vi "骰寶.vi"() -> ()   [LabVIEW 2014]
panel:
  in  "Listbox 2":i32[](listbox)
  in  "Listbox 3":i32[](listbox)
  in  "Listbox":i32[](listbox)
  in  "遊戲開始":bool
  out "總共賺取/賠掉金額":i32
  out "經歷輪數":i32
  out "此輪賺取/賠掉金額":i32
  out "賭金金額":i32
  out "Boolean":T1
  in  "Cluster 7":T2={"Color Box 4"=16448250, "Boolean 5"=FALSE, "Boolean 11"=FALSE, "Boolean 12"=FALSE, "Boolean 13"=FALSE, "Boolean 14"=FALSE, "Boolean 15"=FALSE}
  in  "Cluster 6":T3={"Color Box"=16777215, "Boolean 4"=FALSE, "Boolean 5"=FALSE, "Boolean 6"=FALSE, "Boolean 7"=FALSE, "Boolean 8"=FALSE}
  in  "Cluster 5":T4={"Color Box 2"=16777215, "Boolean 3"=FALSE, "Boolean 4"=FALSE, "Boolean 6"=FALSE, "Boolean 5"=FALSE}
  in  "Cluster 4":T5={"Color Box 2"=16777215, "Boolean"=FALSE, "Boolean 3"=FALSE, "Boolean 2"=FALSE}
  in  "Cluster 3":T6={"Color Box"=16777215, "Boolean"=FALSE, "Boolean 2"=FALSE}
  in  "Cluster 2":T7={"Color Box"=16777215, "Boolean"=FALSE}
  in  "下注金額":i32=10 min=10 max=50
  out "Enum":enum16{"3", "2", "1"}(ring)=enum."2"
  out "骰子點數":i32
  out "比較值3":i32
  out "比較值2":i32
  out "比較值1":i32
  in  "退出比賽":bool
  in  "下好離手":bool
  in  "進行下一輪":bool
  in  "下注盤":T8
  # "遊戲介紹:"
  # "遊戲操作:"
  # "注意事項:"
  # "以上說明都看完沒問題的話，\n就可以按下遊戲開始開始遊玩囉!\n                        ↓"
  # "骰子點數"
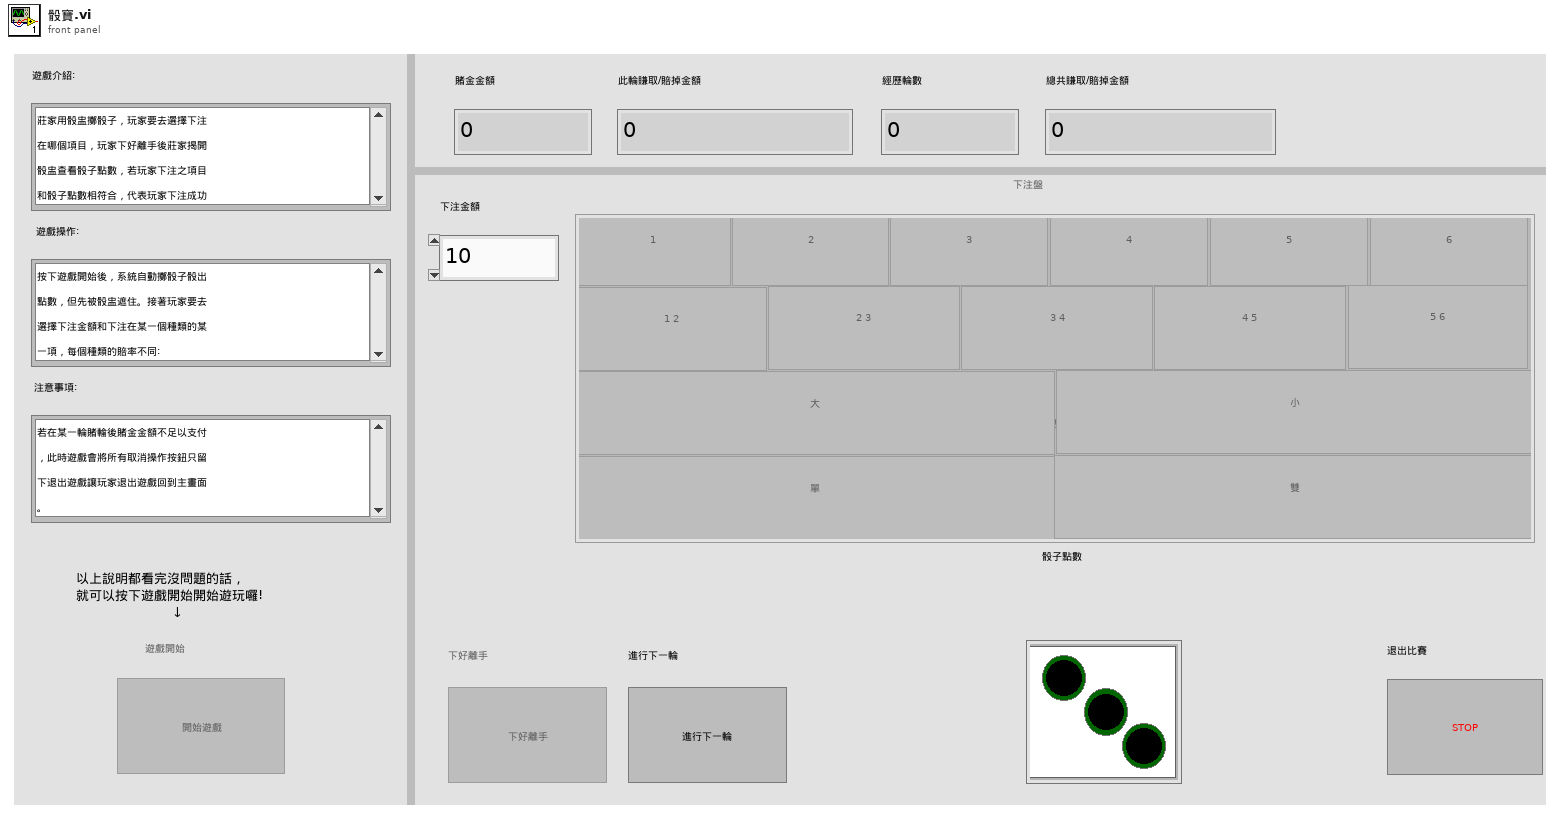
[diagram p1: front panel]
types:
  T1 = typedef "骰盅.ctl" = bool
  T2 = typedef "點數六.ctl" = cluster{"Color Box 4":u32, "Boolean 5":bool, "Boolean 11":bool, "Boolean 12":bool, "Boolean 13":bool, "Boolean 14":bool, "Boolean 15":bool}
  T3 = typedef "き.ctl" = cluster{"Color Box":u32, "Boolean 4":bool, "Boolean 5":bool, "Boolean 6":bool, "Boolean 7":bool, "Boolean 8":bool}
  T4 = typedef "點數四.ctl" = cluster{"Color Box 2":u32, "Boolean 3":bool, "Boolean 4":bool, "Boolean 6":bool, "Boolean 5":bool}
  T5 = typedef "點數三.ctl" = cluster{"Color Box 2":u32, "Boolean":bool, "Boolean 3":bool, "Boolean 2":bool}
  T6 = typedef "點數二.ctl" = cluster{"Color Box":u32, "Boolean":bool, "Boolean 2":bool}
  T7 = typedef "點數一.ctl" = cluster{"Color Box":u32, "Boolean":bool}
  T8 = cluster{" 單":bool, "雙":bool, "大":bool, "小 ":bool, "1 2":bool, "2 3":bool, "3 4":bool, "4 5":bool, "5 6":bool, "1":bool, "2":bool, "3":bool, "4 ":bool, "5":bool, "6":bool}
  T9 = enum16{"restart", "display dice's number and compare 3", "display dice's number and compare 2", "display dice's number and compare 1", "Get out of hand", "player select item", "throw dice(not display)", "wait start button press", "init"}
  T10 = enum8{"Enabled", "Disabled", "Disabled and Grayed Out"}
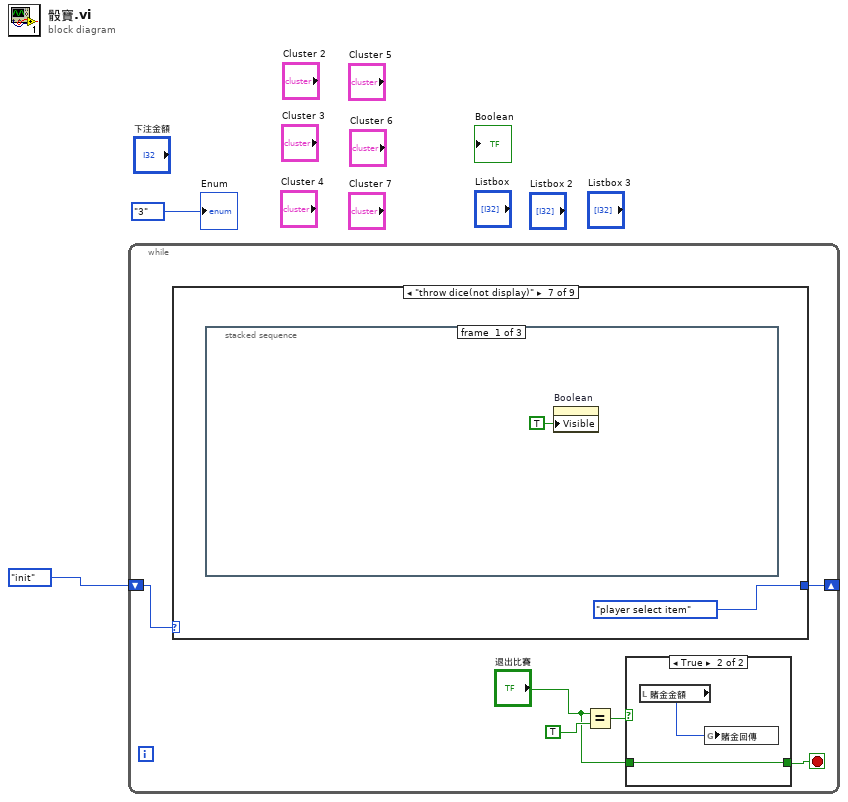
[diagram p0: block diagram]
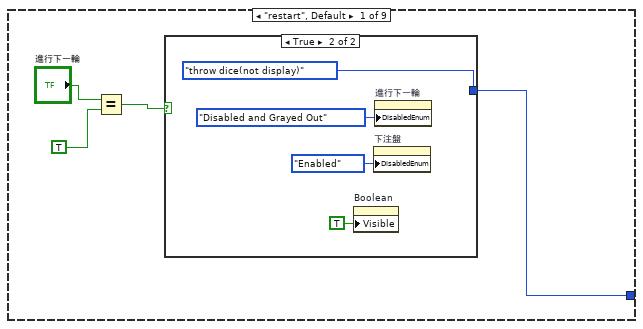
[diagram p3: hidden frame]
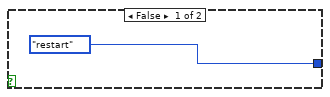
[diagram p4: hidden frame]
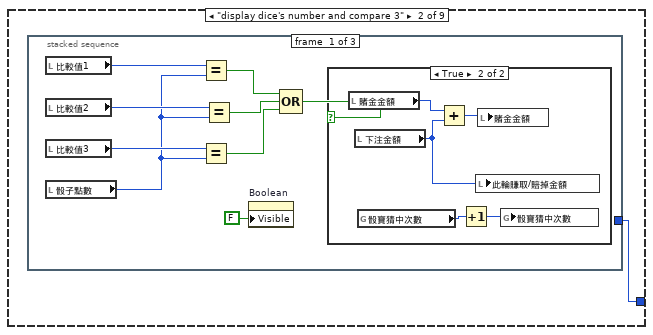
[diagram p5: hidden frame]
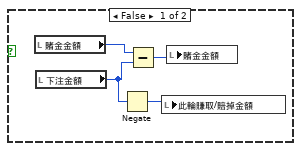
[diagram p6: hidden frame]
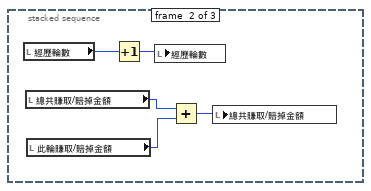
[diagram p7: hidden frame]
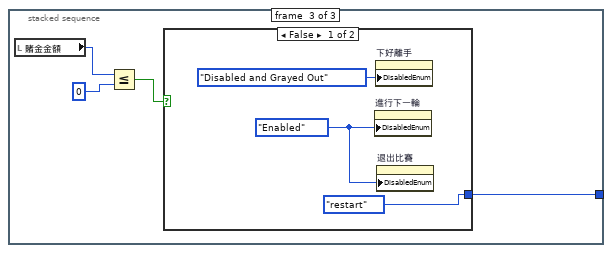
[diagram p8: hidden frame]
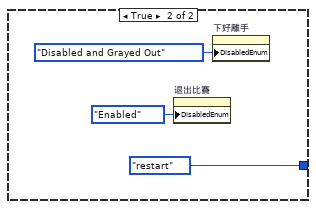
[diagram p9: hidden frame]
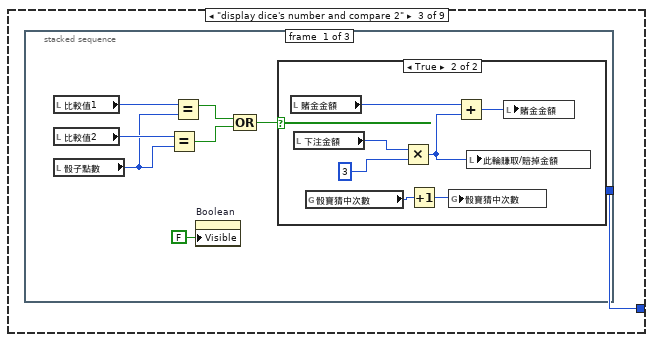
[diagram p10: hidden frame]
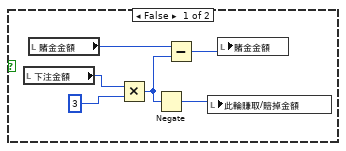
[diagram p11: hidden frame]
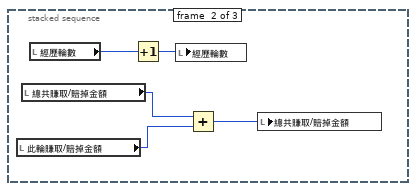
[diagram p12: hidden frame]
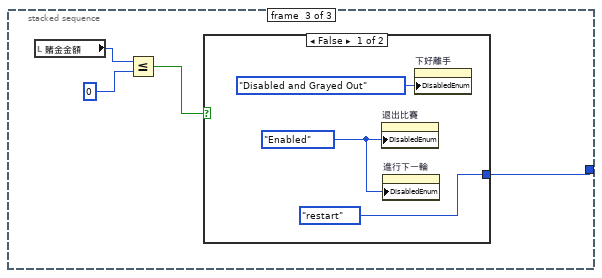
[diagram p13: hidden frame]
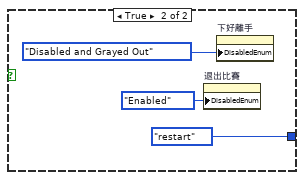
[diagram p14: hidden frame]
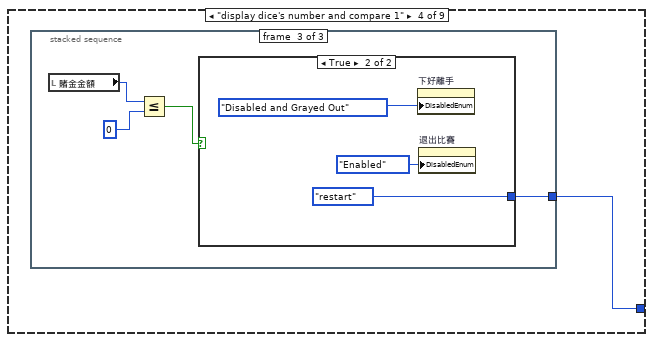
[diagram p15: hidden frame]
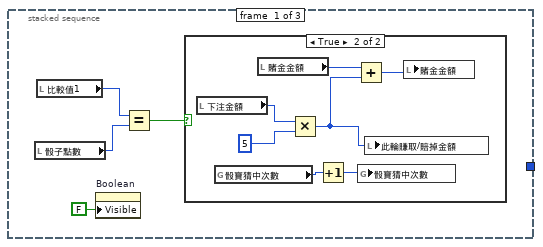
[diagram p16: hidden frame]
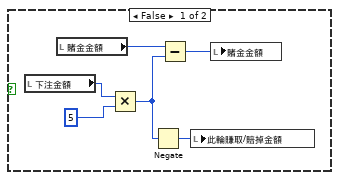
[diagram p17: hidden frame]
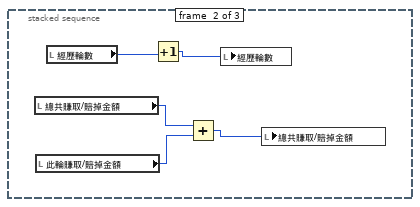
[diagram p18: hidden frame]
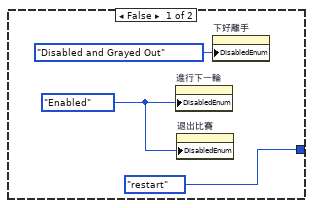
[diagram p19: hidden frame]
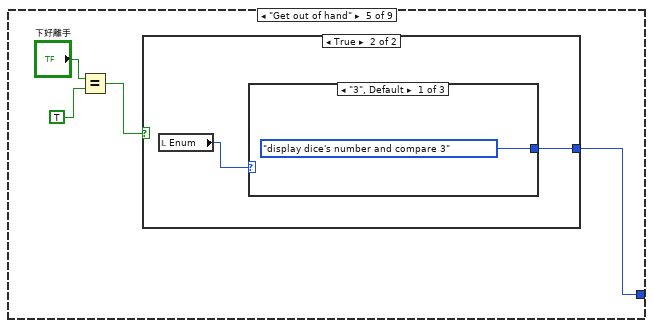
[diagram p20: hidden frame]
diagram:
  n1 = while {
    shift-right: [w7] -> _
    shift-left: T9."init" -> [w8]
    stop <- w3 stop-if-true
    n2 = case shown="\"throw dice(not display)\"" w8 {
      tunnel: [w12 w21 w55 w91 w124 w134 T9."player select item" w249 T9."wait start button press"] -> w7
      frame "restart", Default {
        n3 = Equal?(x="進行下一輪", y=TRUE) -> (x = y?=w15:bool)
        n4 = case shown="True" w15 {
          tunnel: [T9."restart" T9."throw dice(not display)"] -> w12
          frame False {
          }
          frame True {
            n5 = property on="Boolean" class="Bool (strict)"("Visible"=TRUE) -> ()  [unwired: 2 in, 2 out]
            n6 = property on="下注盤" class="Clust"("DisabledEnum"=T10."Enabled" ("Disabled")) -> ()  [unwired: 2 in, 2 out]
            n7 = property on="進行下一輪" class="Bool"("DisabledEnum"=T10."Disabled and Grayed Out" ("Disabled")) -> ()  [unwired: 2 in, 2 out]
          }
        }
      }
      frame "display dice's number and compare 3" {
        n8 = stacked-sequence {
          tunnel: [_ _ w45] -> w21
          frame #0 {
            n9 = local read "比較值1"() -> (w30:i32)
            n10 = local read "比較值2"() -> (w29:i32)
            n11 = local read "比較值3"() -> (w28:i32)
            n12 = local read "骰子點數"() -> (w27:i32)
            n13 = Equal?(x=w30, y=w27) -> (x = y?=w26:bool)
            n14 = Equal?(x=w28, y=w27) -> (x = y?=w24:bool)
            n15 = Equal?(x=w29, y=w27) -> (x = y?=w25:bool)
            n16 = property on="Boolean" class="Bool (strict)"("Visible"=FALSE) -> ()  [unwired: 2 in, 2 out]
            n17 = Compound Arithmetic op=OR(w26, w25, w24) -> (w23:bool)
            n18 = case shown="True" w23 {
              frame False {
                n19 = local read "賭金金額"() -> (w34:i32)
                n20 = local read "下注金額"() -> (w31:i32)
                n21 = Negate(x=w31) -> (-x=w32:i32)
                n22 = Subtract(x=w34, y=w31) -> (x-y=w33:i32)
                n23 = local write "此輪賺取/賠掉金額"(w32) -> ()
                n24 = local write "賭金金額"(w33) -> ()
              }
              frame True {
                n25 = local read "賭金金額"() -> (w39:i32)
                n26 = local read "下注金額"() -> (w37:i32)
                n27 = global read "global variable-骰寶猜中次數.vi" "骰寶猜中次數"() -> (w36:i32)
                n28 = Add(x=w39, y=w37) -> (x+y=w38:i32)
                n29 = Increment(x=w36) -> (x+1=w35:i32)
                n30 = local write "此輪賺取/賠掉金額"(w37) -> ()
                n31 = local write "賭金金額"(w38) -> ()
                n32 = global write "global variable-骰寶猜中次數.vi" "骰寶猜中次數"(w35) -> ()
              }
            }
          }
          frame #1 {
            n33 = local read "經歷輪數"() -> (w44:i32)
            n34 = local read "總共賺取/賠掉金額"() -> (w42:i32)
            n35 = local read "此輪賺取/賠掉金額"() -> (w41:i32)
            n36 = Increment(x=w44) -> (x+1=w43:i32)
            n37 = local write "經歷輪數"(w43) -> ()
            n38 = Add(x=w42, y=w41) -> (x+y=w40:i32)
            n39 = local write "總共賺取/賠掉金額"(w40) -> ()
          }
          frame #2 {
            n40 = local read "賭金金額"() -> (w48:i32)
            n41 = Less Or Equal?(x=w48, y=0) -> (x <= y?=w46:bool)
            n42 = case shown="False" w46 {
              tunnel: [T9."restart" T9."restart"] -> w45
              frame False {
                w50 = T10."Enabled" ("Disabled")
                n43 = property on="進行下一輪" class="Bool"("DisabledEnum"=w50) -> ()  [unwired: 2 in, 2 out]
                n44 = property on="下好離手" class="Bool"("DisabledEnum"=T10."Disabled and Grayed Out" ("Disabled")) -> ()  [unwired: 2 in, 2 out]
                n45 = property on="退出比賽" class="Bool"("DisabledEnum"=w50) -> ()  [unwired: 2 in, 2 out]
              }
              frame True {
                n46 = property on="退出比賽" class="Bool"("DisabledEnum"=T10."Enabled" ("Disabled")) -> ()  [unwired: 2 in, 2 out]
                n47 = property on="下好離手" class="Bool"("DisabledEnum"=T10."Disabled and Grayed Out" ("Disabled")) -> ()  [unwired: 2 in, 2 out]
              }
            }
          }
        }
      }
      frame "display dice's number and compare 2" {
        n48 = stacked-sequence {
          tunnel: [_ _ w81] -> w55
          frame #0 {
            n49 = local read "比較值1"() -> (w62:i32)
            n50 = local read "比較值2"() -> (w61:i32)
            n51 = local read "骰子點數"() -> (w60:i32)
            n52 = Equal?(x=w61, y=w60) -> (x = y?=w58:bool)
            n53 = Equal?(x=w62, y=w60) -> (x = y?=w59:bool)
            n54 = property on="Boolean" class="Bool (strict)"("Visible"=FALSE) -> ()  [unwired: 2 in, 2 out]
            n55 = Compound Arithmetic op=OR(w59, w58) -> (w57:bool)
            n56 = case shown="True" w57 {
              frame False {
                n57 = local read "下注金額"() -> (w68:i32)
                n58 = local read "賭金金額"() -> (w66:i32)
                n59 = Multiply(x=w68, y=3) -> (x*y=w63:i32)
                n60 = Negate(x=w63) -> (-x=w64:i32)
                n61 = Subtract(x=w66, y=w63) -> (x-y=w65:i32)
                n62 = local write "此輪賺取/賠掉金額"(w64) -> ()
                n63 = local write "賭金金額"(w65) -> ()
              }
              frame True {
                n64 = local read "賭金金額"() -> (w73:i32)
                n65 = local read "下注金額"() -> (w75:i32)
                n66 = global read "global variable-骰寶猜中次數.vi" "骰寶猜中次數"() -> (w69:i32)
                n67 = Multiply(x=w75, y=3) -> (x*y=w71:i32)
                n68 = Increment(x=w69) -> (x+1=w70:i32)
                n69 = global write "global variable-骰寶猜中次數.vi" "骰寶猜中次數"(w70) -> ()
                n70 = Add(x=w73, y=w71) -> (x+y=w72:i32)
                n71 = local write "此輪賺取/賠掉金額"(w71) -> ()
                n72 = local write "賭金金額"(w72) -> ()
              }
            }
          }
          frame #1 {
            n73 = local read "此輪賺取/賠掉金額"() -> (w77:i32)
            n74 = local read "總共賺取/賠掉金額"() -> (w78:i32)
            n75 = local read "經歷輪數"() -> (w80:i32)
            n76 = Increment(x=w80) -> (x+1=w79:i32)
            n77 = local write "經歷輪數"(w79) -> ()
            n78 = Add(x=w78, y=w77) -> (x+y=w76:i32)
            n79 = local write "總共賺取/賠掉金額"(w76) -> ()
          }
          frame #2 {
            n80 = local read "賭金金額"() -> (w84:i32)
            n81 = Less Or Equal?(x=w84, y=0) -> (x <= y?=w82:bool)
            n82 = case shown="False" w82 {
              tunnel: [T9."restart" T9."restart"] -> w81
              frame False {
                w87 = T10."Enabled" ("Disabled")
                n83 = property on="退出比賽" class="Bool"("DisabledEnum"=w87) -> ()  [unwired: 2 in, 2 out]
                n84 = property on="進行下一輪" class="Bool"("DisabledEnum"=w87) -> ()  [unwired: 2 in, 2 out]
                n85 = property on="下好離手" class="Bool"("DisabledEnum"=T10."Disabled and Grayed Out" ("Disabled")) -> ()  [unwired: 2 in, 2 out]
              }
              frame True {
                n86 = property on="退出比賽" class="Bool"("DisabledEnum"=T10."Enabled" ("Disabled")) -> ()  [unwired: 2 in, 2 out]
                n87 = property on="下好離手" class="Bool"("DisabledEnum"=T10."Disabled and Grayed Out" ("Disabled")) -> ()  [unwired: 2 in, 2 out]
              }
            }
          }
        }
      }
      frame "display dice's number and compare 1" {
        n88 = stacked-sequence {
          tunnel: [_ _ w114] -> w91
          frame #0 {
            n89 = local read "骰子點數"() -> (w95:i32)
            n90 = local read "比較值1"() -> (w94:i32)
            n91 = property on="Boolean" class="Bool (strict)"("Visible"=FALSE) -> ()  [unwired: 2 in, 2 out]
            n92 = Equal?(x=w94, y=w95) -> (x = y?=w93:bool)
            n93 = case shown="True" w93 {
              frame False {
                n94 = local read "下注金額"() -> (w101:i32)
                n95 = local read "賭金金額"() -> (w99:i32)
                n96 = Multiply(x=w101, y=5) -> (x*y=w96:i32)
                n97 = Negate(x=w96) -> (-x=w97:i32)
                n98 = Subtract(x=w99, y=w96) -> (x-y=w98:i32)
                n99 = local write "此輪賺取/賠掉金額"(w97) -> ()
                n100 = local write "賭金金額"(w98) -> ()
              }
              frame True {
                n101 = local read "下注金額"() -> (w108:i32)
                n102 = global read "global variable-骰寶猜中次數.vi" "骰寶猜中次數"() -> (w102:i32)
                n103 = local read "賭金金額"() -> (w106:i32)
                n104 = Multiply(x=w108, y=5) -> (x*y=w104:i32)
                n105 = Increment(x=w102) -> (x+1=w103:i32)
                n106 = Add(x=w106, y=w104) -> (x+y=w105:i32)
                n107 = global write "global variable-骰寶猜中次數.vi" "骰寶猜中次數"(w103) -> ()
                n108 = local write "此輪賺取/賠掉金額"(w104) -> ()
                n109 = local write "賭金金額"(w105) -> ()
              }
            }
          }
          frame #1 {
            n110 = local read "總共賺取/賠掉金額"() -> (w111:i32)
            n111 = local read "此輪賺取/賠掉金額"() -> (w110:i32)
            n112 = local read "經歷輪數"() -> (w113:i32)
            n113 = Increment(x=w113) -> (x+1=w112:i32)
            n114 = Add(x=w111, y=w110) -> (x+y=w109:i32)
            n115 = local write "經歷輪數"(w112) -> ()
            n116 = local write "總共賺取/賠掉金額"(w109) -> ()
          }
          frame #2 {
            n117 = local read "賭金金額"() -> (w117:i32)
            n118 = Less Or Equal?(x=w117, y=0) -> (x <= y?=w115:bool)
            n119 = case shown="True" w115 {
              tunnel: [T9."restart" T9."restart"] -> w114
              frame False {
                w120 = T10."Enabled" ("Disabled")
                n120 = property on="進行下一輪" class="Bool"("DisabledEnum"=w120) -> ()  [unwired: 2 in, 2 out]
                n121 = property on="退出比賽" class="Bool"("DisabledEnum"=w120) -> ()  [unwired: 2 in, 2 out]
                n122 = property on="下好離手" class="Bool"("DisabledEnum"=T10."Disabled and Grayed Out" ("Disabled")) -> ()  [unwired: 2 in, 2 out]
              }
              frame True {
                n123 = property on="下好離手" class="Bool"("DisabledEnum"=T10."Disabled and Grayed Out" ("Disabled")) -> ()  [unwired: 2 in, 2 out]
                n124 = property on="退出比賽" class="Bool"("DisabledEnum"=T10."Enabled" ("Disabled")) -> ()  [unwired: 2 in, 2 out]
              }
            }
          }
        }
      }
      frame "Get out of hand" {
        n125 = Equal?(x="下好離手", y=TRUE) -> (x = y?=w126:bool)
        n126 = case shown="True" w126 {
          tunnel: [T9."Get out of hand" w129] -> w124
          frame False {
          }
          frame True {
            n127 = local read "Enum"() -> (w130:enum16{"3", "2", "1"})
            n128 = case shown="\"3\", Default" w130 {
              tunnel: [T9."display dice's number and compare 3" T9."display dice's number and compare 2" T9."display dice's number and compare 1"] -> w129
              frame "3", Default {
              }
              frame "2" {
              }
              frame "1" {
              }
            }
          }
        }
      }
      frame "player select item" {
        n129 = Cluster To Array(cluster="下注盤") -> (array=w136:bool[])
        n130 = Search 1D Array(1D array=w136, element=TRUE) -> (index of element=w138:i32)  [unwired: 1 in]
        n131 = case shown="0" w138 {
          tunnel: [T9."player select item" T9."Get out of hand" T9."Get out of hand" T9."Get out of hand" T9."Get out of hand" T9."Get out of hand" T9."Get out of hand" T9."Get out of hand" T9."Get out of hand" T9."Get out of hand" T9."Get out of hand" T9."Get out of hand" T9."Get out of hand" T9."Get out of hand" T9."Get out of hand" T9."Get out of hand"] -> w134
          frame -1, Default {
          }
          frame 0 {
            n132 = local write "比較值2"(3 ("比較值2")) -> ()
            n133 = local write "比較值3"(5 ("比較值3")) -> ()
            n134 = local write "比較值1"(1) -> ()
            n135 = local write "Enum"(enum16{"3", "2", "1"}."3" ("Enum")) -> ()
            n136 = property on="下好離手" class="Bool"("DisabledEnum"=T10."Enabled" ("Disabled")) -> ()  [unwired: 2 in, 2 out]
            n137 = property on="下注盤" class="Clust"("DisabledEnum"=T10."Disabled and Grayed Out" ("Disabled")) -> ()  [unwired: 2 in, 2 out]
          }
          frame 1 {
            n138 = local write "比較值3"(6 ("比較值3")) -> ()
            n139 = local write "比較值2"(4 ("比較值2")) -> ()
            n140 = local write "比較值1"(2 ("比較值1")) -> ()
            n141 = local write "Enum"(enum16{"3", "2", "1"}."3" ("Enum")) -> ()
            n142 = property on="下好離手" class="Bool"("DisabledEnum"=T10."Enabled" ("Disabled")) -> ()  [unwired: 2 in, 2 out]
            n143 = property on="下注盤" class="Clust"("DisabledEnum"=T10."Disabled and Grayed Out" ("Disabled")) -> ()  [unwired: 2 in, 2 out]
          }
          frame 2 {
            n144 = local write "比較值3"(4 ("比較值3")) -> ()
            n145 = local write "比較值1"(6 ("比較值1")) -> ()
            n146 = local write "比較值2"(5 ("比較值2")) -> ()
            n147 = local write "Enum"(enum16{"3", "2", "1"}."3" ("Enum")) -> ()
            n148 = property on="下好離手" class="Bool"("DisabledEnum"=T10."Enabled" ("Disabled")) -> ()  [unwired: 2 in, 2 out]
            n149 = property on="下注盤" class="Clust"("DisabledEnum"=T10."Disabled and Grayed Out" ("Disabled")) -> ()  [unwired: 2 in, 2 out]
          }
          frame 3 {
            n150 = local write "比較值2"(2 ("比較值2")) -> ()
            n151 = local write "比較值3"(1 ("比較值3")) -> ()
            n152 = local write "比較值1"(3 ("比較值1")) -> ()
            n153 = local write "Enum"(enum16{"3", "2", "1"}."3" ("Enum")) -> ()
            n154 = property on="下好離手" class="Bool"("DisabledEnum"=T10."Enabled" ("Disabled")) -> ()  [unwired: 2 in, 2 out]
            n155 = property on="下注盤" class="Clust"("DisabledEnum"=T10."Disabled and Grayed Out" ("Disabled")) -> ()  [unwired: 2 in, 2 out]
          }
          frame 4 {
            n156 = local write "比較值1"(1 ("比較值1")) -> ()
            n157 = local write "比較值2"(2 ("比較值2")) -> ()
            n158 = local write "Enum"(enum16{"3", "2", "1"}."2" ("Enum")) -> ()
            n159 = property on="下好離手" class="Bool"("DisabledEnum"=T10."Enabled" ("Disabled")) -> ()  [unwired: 2 in, 2 out]
            n160 = property on="下注盤" class="Clust"("DisabledEnum"=T10."Disabled and Grayed Out" ("Disabled")) -> ()  [unwired: 2 in, 2 out]
          }
          frame 5 {
            n161 = local write "比較值1"(2 ("比較值1")) -> ()
            n162 = local write "比較值2"(3 ("比較值2")) -> ()
            n163 = local write "Enum"(enum16{"3", "2", "1"}."2" ("Enum")) -> ()
            n164 = property on="下好離手" class="Bool"("DisabledEnum"=T10."Enabled" ("Disabled")) -> ()  [unwired: 2 in, 2 out]
            n165 = property on="下注盤" class="Clust"("DisabledEnum"=T10."Disabled and Grayed Out" ("Disabled")) -> ()  [unwired: 2 in, 2 out]
          }
          frame 6 {
            n166 = local write "比較值1"(3 ("比較值1")) -> ()
            n167 = local write "比較值2"(4 ("比較值2")) -> ()
            n168 = local write "Enum"(enum16{"3", "2", "1"}."2" ("Enum")) -> ()
            n169 = property on="下好離手" class="Bool"("DisabledEnum"=T10."Enabled" ("Disabled")) -> ()  [unwired: 2 in, 2 out]
            n170 = property on="下注盤" class="Clust"("DisabledEnum"=T10."Disabled and Grayed Out" ("Disabled")) -> ()  [unwired: 2 in, 2 out]
          }
          frame 7 {
            n171 = local write "比較值1"(4 ("比較值1")) -> ()
            n172 = local write "比較值2"(5 ("比較值2")) -> ()
            n173 = local write "Enum"(enum16{"3", "2", "1"}."2" ("Enum")) -> ()
            n174 = property on="下好離手" class="Bool"("DisabledEnum"=T10."Enabled" ("Disabled")) -> ()  [unwired: 2 in, 2 out]
            n175 = property on="下注盤" class="Clust"("DisabledEnum"=T10."Disabled and Grayed Out" ("Disabled")) -> ()  [unwired: 2 in, 2 out]
          }
          frame 8 {
            n176 = local write "比較值2"(6 ("比較值2")) -> ()
            n177 = local write "比較值1"(5 ("比較值1")) -> ()
            n178 = local write "Enum"(enum16{"3", "2", "1"}."2" ("Enum")) -> ()
            n179 = property on="下好離手" class="Bool"("DisabledEnum"=T10."Enabled" ("Disabled")) -> ()  [unwired: 2 in, 2 out]
            n180 = property on="下注盤" class="Clust"("DisabledEnum"=T10."Disabled and Grayed Out" ("Disabled")) -> ()  [unwired: 2 in, 2 out]
          }
          frame 9 {
            n181 = local write "比較值1"(1 ("比較值1")) -> ()
            n182 = local write "Enum"(enum16{"3", "2", "1"}."1" ("Enum")) -> ()
            n183 = property on="下好離手" class="Bool"("DisabledEnum"=T10."Enabled" ("Disabled")) -> ()  [unwired: 2 in, 2 out]
            n184 = property on="下注盤" class="Clust"("DisabledEnum"=T10."Disabled and Grayed Out" ("Disabled")) -> ()  [unwired: 2 in, 2 out]
          }
          frame 10 {
            n185 = local write "比較值1"(2 ("比較值1")) -> ()
            n186 = local write "Enum"(enum16{"3", "2", "1"}."1" ("Enum")) -> ()
            n187 = property on="下好離手" class="Bool"("DisabledEnum"=T10."Enabled" ("Disabled")) -> ()  [unwired: 2 in, 2 out]
            n188 = property on="下注盤" class="Clust"("DisabledEnum"=T10."Disabled and Grayed Out" ("Disabled")) -> ()  [unwired: 2 in, 2 out]
          }
          frame 11 {
            n189 = local write "比較值1"(3 ("比較值1")) -> ()
            n190 = local write "Enum"(enum16{"3", "2", "1"}."1" ("Enum")) -> ()
            n191 = property on="下好離手" class="Bool"("DisabledEnum"=T10."Enabled" ("Disabled")) -> ()  [unwired: 2 in, 2 out]
            n192 = property on="下注盤" class="Clust"("DisabledEnum"=T10."Disabled and Grayed Out" ("Disabled")) -> ()  [unwired: 2 in, 2 out]
          }
          frame 12 {
            n193 = local write "比較值1"(4 ("比較值1")) -> ()
            n194 = local write "Enum"(enum16{"3", "2", "1"}."1" ("Enum")) -> ()
            n195 = property on="下好離手" class="Bool"("DisabledEnum"=T10."Enabled" ("Disabled")) -> ()  [unwired: 2 in, 2 out]
            n196 = property on="下注盤" class="Clust"("DisabledEnum"=T10."Disabled and Grayed Out" ("Disabled")) -> ()  [unwired: 2 in, 2 out]
          }
          frame 13 {
            n197 = local write "比較值1"(5 ("比較值1")) -> ()
            n198 = local write "Enum"(enum16{"3", "2", "1"}."1" ("Enum")) -> ()
            n199 = property on="下好離手" class="Bool"("DisabledEnum"=T10."Enabled" ("Disabled")) -> ()  [unwired: 2 in, 2 out]
            n200 = property on="下注盤" class="Clust"("DisabledEnum"=T10."Disabled and Grayed Out" ("Disabled")) -> ()  [unwired: 2 in, 2 out]
          }
          frame 14 {
            n201 = local write "比較值1"(6 ("比較值1")) -> ()
            n202 = local write "Enum"(enum16{"3", "2", "1"}."1" ("Enum")) -> ()
            n203 = property on="下好離手" class="Bool"("DisabledEnum"=T10."Enabled" ("Disabled")) -> ()  [unwired: 2 in, 2 out]
            n204 = property on="下注盤" class="Clust"("DisabledEnum"=T10."Disabled and Grayed Out" ("Disabled")) -> ()  [unwired: 2 in, 2 out]
          }
        }
      }
      frame "throw dice(not display)" {
        n205 = stacked-sequence {
          frame #0 {
            n206 = property on="Boolean" class="Bool (strict)"("Visible"=TRUE) -> ()  [unwired: 2 in, 2 out]
          }
          frame #1 {
            n207 = Random Number (0-1)() -> (number: 0 to 1=w235:dbl)
            n208 = Multiply(x=w235, y=6.0) -> (x*y=w233:dbl)
            n209 = Add(x=w233, y=0.5) -> (x+y=w231:dbl)
            n210 = To Long Integer(number=w231) -> (32bit integer=w230:i32)
            n211 = local write "骰子點數"(w230) -> ()
            n212 = case shown="6" w230 {
              frame 1, Default {
                w236 = FALSE
                n213 = property on="Cluster 3" class="Clust (strict)"("Visible"=w236) -> ()  [unwired: 2 in, 2 out]
                n214 = property on="Cluster 4" class="Clust (strict)"("Visible"=w236) -> ()  [unwired: 2 in, 2 out]
                n215 = property on="Cluster 2" class="Clust (strict)"("Visible"=TRUE) -> ()  [unwired: 2 in, 2 out]
                n216 = property on="Cluster 5" class="Clust (strict)"("Visible"=w236) -> ()  [unwired: 2 in, 2 out]
                n217 = property on="Cluster 6" class="Clust (strict)"("Visible"=w236) -> ()  [unwired: 2 in, 2 out]
                n218 = property on="Cluster 7" class="Clust (strict)"("Visible"=w236) -> ()  [unwired: 2 in, 2 out]
              }
              frame 2 {
                w238 = FALSE
                n219 = property on="Cluster 2" class="Clust (strict)"("Visible"=w238) -> ()  [unwired: 2 in, 2 out]
                n220 = property on="Cluster 4" class="Clust (strict)"("Visible"=w238) -> ()  [unwired: 2 in, 2 out]
                n221 = property on="Cluster 3" class="Clust (strict)"("Visible"=TRUE) -> ()  [unwired: 2 in, 2 out]
                n222 = property on="Cluster 5" class="Clust (strict)"("Visible"=w238) -> ()  [unwired: 2 in, 2 out]
                n223 = property on="Cluster 6" class="Clust (strict)"("Visible"=w238) -> ()  [unwired: 2 in, 2 out]
                n224 = property on="Cluster 7" class="Clust (strict)"("Visible"=w238) -> ()  [unwired: 2 in, 2 out]
              }
              frame 3 {
                w240 = FALSE
                n225 = property on="Cluster 2" class="Clust (strict)"("Visible"=w240) -> ()  [unwired: 2 in, 2 out]
                n226 = property on="Cluster 4" class="Clust (strict)"("Visible"=TRUE) -> ()  [unwired: 2 in, 2 out]
                n227 = property on="Cluster 3" class="Clust (strict)"("Visible"=w240) -> ()  [unwired: 2 in, 2 out]
                n228 = property on="Cluster 5" class="Clust (strict)"("Visible"=w240) -> ()  [unwired: 2 in, 2 out]
                n229 = property on="Cluster 7" class="Clust (strict)"("Visible"=w240) -> ()  [unwired: 2 in, 2 out]
                n230 = property on="Cluster 6" class="Clust (strict)"("Visible"=w240) -> ()  [unwired: 2 in, 2 out]
              }
              frame 4 {
                w242 = FALSE
                n231 = property on="Cluster 5" class="Clust (strict)"("Visible"=TRUE) -> ()  [unwired: 2 in, 2 out]
                n232 = property on="Cluster 3" class="Clust (strict)"("Visible"=w242) -> ()  [unwired: 2 in, 2 out]
                n233 = property on="Cluster 2" class="Clust (strict)"("Visible"=w242) -> ()  [unwired: 2 in, 2 out]
                n234 = property on="Cluster 4" class="Clust (strict)"("Visible"=w242) -> ()  [unwired: 2 in, 2 out]
                n235 = property on="Cluster 6" class="Clust (strict)"("Visible"=w242) -> ()  [unwired: 2 in, 2 out]
                n236 = property on="Cluster 7" class="Clust (strict)"("Visible"=w242) -> ()  [unwired: 2 in, 2 out]
              }
              frame 5 {
                w244 = FALSE
                n237 = property on="Cluster 2" class="Clust (strict)"("Visible"=w244) -> ()  [unwired: 2 in, 2 out]
                n238 = property on="Cluster 3" class="Clust (strict)"("Visible"=w244) -> ()  [unwired: 2 in, 2 out]
                n239 = property on="Cluster 4" class="Clust (strict)"("Visible"=w244) -> ()  [unwired: 2 in, 2 out]
                n240 = property on="Cluster 6" class="Clust (strict)"("Visible"=TRUE) -> ()  [unwired: 2 in, 2 out]
                n241 = property on="Cluster 5" class="Clust (strict)"("Visible"=w244) -> ()  [unwired: 2 in, 2 out]
                n242 = property on="Cluster 7" class="Clust (strict)"("Visible"=w244) -> ()  [unwired: 2 in, 2 out]
              }
              frame 6 {
                w246 = FALSE
                n243 = property on="Cluster 4" class="Clust (strict)"("Visible"=w246) -> ()  [unwired: 2 in, 2 out]
                n244 = property on="Cluster 3" class="Clust (strict)"("Visible"=w246) -> ()  [unwired: 2 in, 2 out]
                n245 = property on="Cluster 2" class="Clust (strict)"("Visible"=w246) -> ()  [unwired: 2 in, 2 out]
                n246 = property on="Cluster 7" class="Clust (strict)"("Visible"=TRUE) -> ()  [unwired: 2 in, 2 out]
                n247 = property on="Cluster 5" class="Clust (strict)"("Visible"=w246) -> ()  [unwired: 2 in, 2 out]
                n248 = property on="Cluster 6" class="Clust (strict)"("Visible"=w246) -> ()  [unwired: 2 in, 2 out]
              }
            }
          }
          frame #2 {
            n249 = One Button Dialog(message="已骰好骰子，請玩家押注") -> ()  [unwired: 1 in, 1 out]
          }
        }
      }
      frame "wait start button press" {
        n250 = Equal?(x="遊戲開始", y=TRUE) -> (x = y?=w252:bool)
        n251 = case shown="False" w252 {
          tunnel: [T9."wait start button press" T9."throw dice(not display)"] -> w249
          frame False {
          }
          frame True {
            w255 = T10."Disabled and Grayed Out" ("Disabled")
            n252 = property on="下注盤" class="Clust"("DisabledEnum"=T10."Enabled" ("Disabled")) -> ()  [unwired: 2 in, 2 out]
            n253 = property on="退出比賽" class="Bool"("DisabledEnum"=w255) -> ()  [unwired: 2 in, 2 out]
            n254 = property on="遊戲開始" class="Bool"("DisabledEnum"=w255) -> ()  [unwired: 2 in, 2 out]
          }
        }
      }
      frame "init" {
        w258 = T10."Disabled and Grayed Out" ("Disabled")
        w262 = 0
        n255 = global read "global variable-賭金金額.vi" "賭金金額"() -> (→"賭金金額":i32)
        n256 = property on="下好離手" class="Bool"("DisabledEnum"=w258) -> ()  [unwired: 2 in, 2 out]
        n257 = property on="進行下一輪" class="Bool"("DisabledEnum"=w258) -> ()  [unwired: 2 in, 2 out]
        n258 = property on="下注盤" class="Clust"("DisabledEnum"=w258) -> ()  [unwired: 2 in, 2 out]
        n259 = property on="遊戲開始" class="Bool"("DisabledEnum"=T10."Enabled" ("Disabled")) -> ()  [unwired: 2 in, 2 out]
        n260 = One Button Dialog(message="歡迎遊玩骰寶，在開始遊戲之前請先詳細閱讀左邊的遊戲說明") -> ()  [unwired: 1 in, 1 out]
        "此輪賺取/賠掉金額" <- w262
        "經歷輪數" <- w262
        "總共賺取/賠掉金額" <- w262
        "比較值2" <- w262
        "比較值1" <- w262
        "骰子點數" <- w262
        "比較值3" <- w262
      }
    }
    n261 = Equal?(x="退出比賽", y=TRUE) -> (x = y?=w5:bool)
    n262 = case shown="True" w5 {
      tunnel: "退出比賽" -> [w9 w11]
      tunnel: [w9 w11] -> w3
      frame False {
      }
      frame True {
        n263 = local read "賭金金額"() -> (w10:i32)
        n264 = global write "global variable-賭金回傳.vi" "賭金回傳"(w10) -> ()
      }
    }
  }
  "Enum" <- enum16{"3", "2", "1"}."3" ("Enum")
